vi "Periodic Tasks.vi"(8 "error in":errorcluster) -> ()   [LabVIEW 2017]
doc: "This VI runs in parallel to other tasks. It can contain as many user-defined periodic loops as you need. These can carry out PID or other sorts of timed response."
uses:
  <vilib>/Rock Robotics/WPI/DriverStation/WPI_DriverStationRobotMode2.ctl
  <vilib>/Rock Robotics/WPI/Utilities/WPI_GetSetVariantRefNum.vi
  Robot Global Data.vi
  <vilib>/Rock Robotics/Network Tables/NT Write Number.vi
panel:
  out "raw yaw":dbl
  out "original Heading":dbl
  out "ignore":dbl
  out "fused":dbl
  out "new yaw":dbl
  in  "Cluster":T1
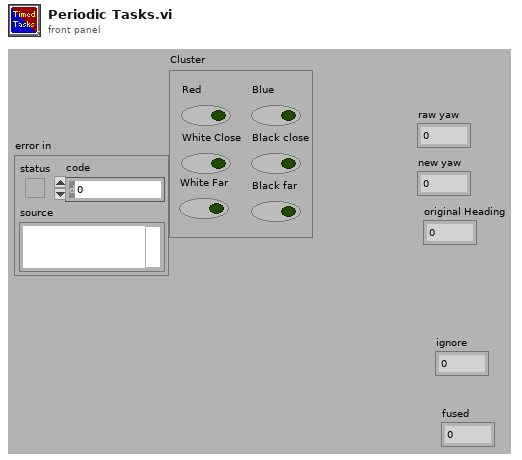
[diagram p1: front panel]
types:
  T1 = cluster{"Red":bool, "Blue":bool, "Black close":bool, "White Close":bool, "White Far":bool, "Black far":bool}
  T2 = typedef "WPI_JoystickDevRef.ctl" = cluster{"Device":T3}
  T3 = typedef "WPI_JoystickDeviceEnum.ctl" = enum16{"USB 0", "USB 1", "USB 2", "USB 3", "USB 4", "USB 5"}
  T4 = typedef "WPI_RobotDriveDevRef.ctl" = cluster{"DevStatus":errorcluster, "Motors[]":T5[], "Square Inputs":bool, "Max Output":dbl}
  T5 = typedef "WPI_MotorControlDeviceRef.ctl" = cluster{"DeviceStatus":errorcluster, "Type":T6, "PWM":cluster{"PWM Channel":T7, "DeadBand":T8}, "CAN":cluster{"Device Number":u8, "SetOutput VI Ref":variant, "GetOutput VI Ref":variant, "Enable VI Ref":variant, "Disable VI Ref":variant, "Data":variant}, "Invert":bool, "DIO PWM":cluster{"PWM \"Enable\" Channel":T7, "DIOChannel":T9, "PWM Rate":dbl}}
  T6 = typedef "WPI_MotorControlType.ctl" = enum16{"PWM", "CAN", "DIO PWM"}
  T7 = typedef "FPGA_DIOPWMChannel.ctl" = enum8{"PWM 0", "PWM 1", "PWM 2", "PWM 3", "PWM 4", "PWM 5", "PWM 6", "PWM 7", "PWM 8", "PWM 9", "PWM MXP 0", "PWM MXP 1", "PWM MXP 2", "PWM MXP 3", "PWM MXP 4", "PWM MXP 5", "PWM MXP 6", "PWM MXP 7", "PWM MXP 8", "PWM MXP 9", "Invalid"}
  T8 = typedef "WPI_PWMDeadband.ctl" = cluster{"Name":string, "maxPositivePwm":i32, "minPositivePwm":i32, "centerPwm":i32, "maxNegativePwm":i32, "minNegativePwm":i32, "angularRange":u16}
  T9 = typedef "FPGA_DIOChannel.ctl" = enum8{"DIO 0", "DIO 1", "DIO 2", "DIO 3", "DIO 4", "DIO 5", "DIO 6", "DIO 7", "DIO 8", "DIO 9", "DIO MXP 0", "DIO MXP 1", "DIO MXP 2", "DIO MXP 3", "DIO MXP 4", "DIO MXP 5", "DIO MXP 6", "DIO MXP 7", "DIO MXP 8", "DIO MXP 9", "DIO MXP 10", "DIO MXP 11", "DIO MXP 12", "DIO MXP 13", "DIO MXP 14", "DIO MXP 15", "SPI Port CS1", "SPI Port CS2", "SPI Port CS3", "SPI Port MISO", "SPI Port MOSI", "Invalid"}
  T10 = typedef "WPI_DriverStationRobotMode2.ctl" = enum16{"Autonomous Disabled", "Autonomous Enabled", "Teleop Disabled", "Teleop Enabled", "Disconnected", "Finish", "Test Disabled", "Test Enabled", "Emergency Stopped"}
  T11 = cluster{"Yaw":dbl, "Roll":dbl, "Pitch":dbl, "Heading":dbl, "Fused Heading":dbl}
  T12 = cluster{"JoystickDevRef":T2, "RobotDriveDevRef":T4}
  T13 = typedef "WPI_EncoderDevRef.ctl" = cluster{"DevStatus":errorcluster, "EncoderIndex":T14, "CounterIndex":T15, "DistancePerCount":dbl, "Decoding Type":T16}
  T14 = typedef "FPGA_EncoderIdx.ctl" = enum8{"Enc 0", "Enc 1", "Enc 2", "Enc 3", "Enc 4", "Enc 5", "Enc 6", "Enc 7", "Invalid"}
  T15 = typedef "FPGA_CounterCtrSystemIndex.ctl" = enum8{"Ctr 0", "Ctr 1", "Ctr 2", "Ctr 3", "Ctr 4", "Ctr 5", "Ctr 6", "Ctr 7", "Invalid"}
  T16 = typedef "WPI_EncoderType.ctl" = enum16{"1x", "2x", "4x"}
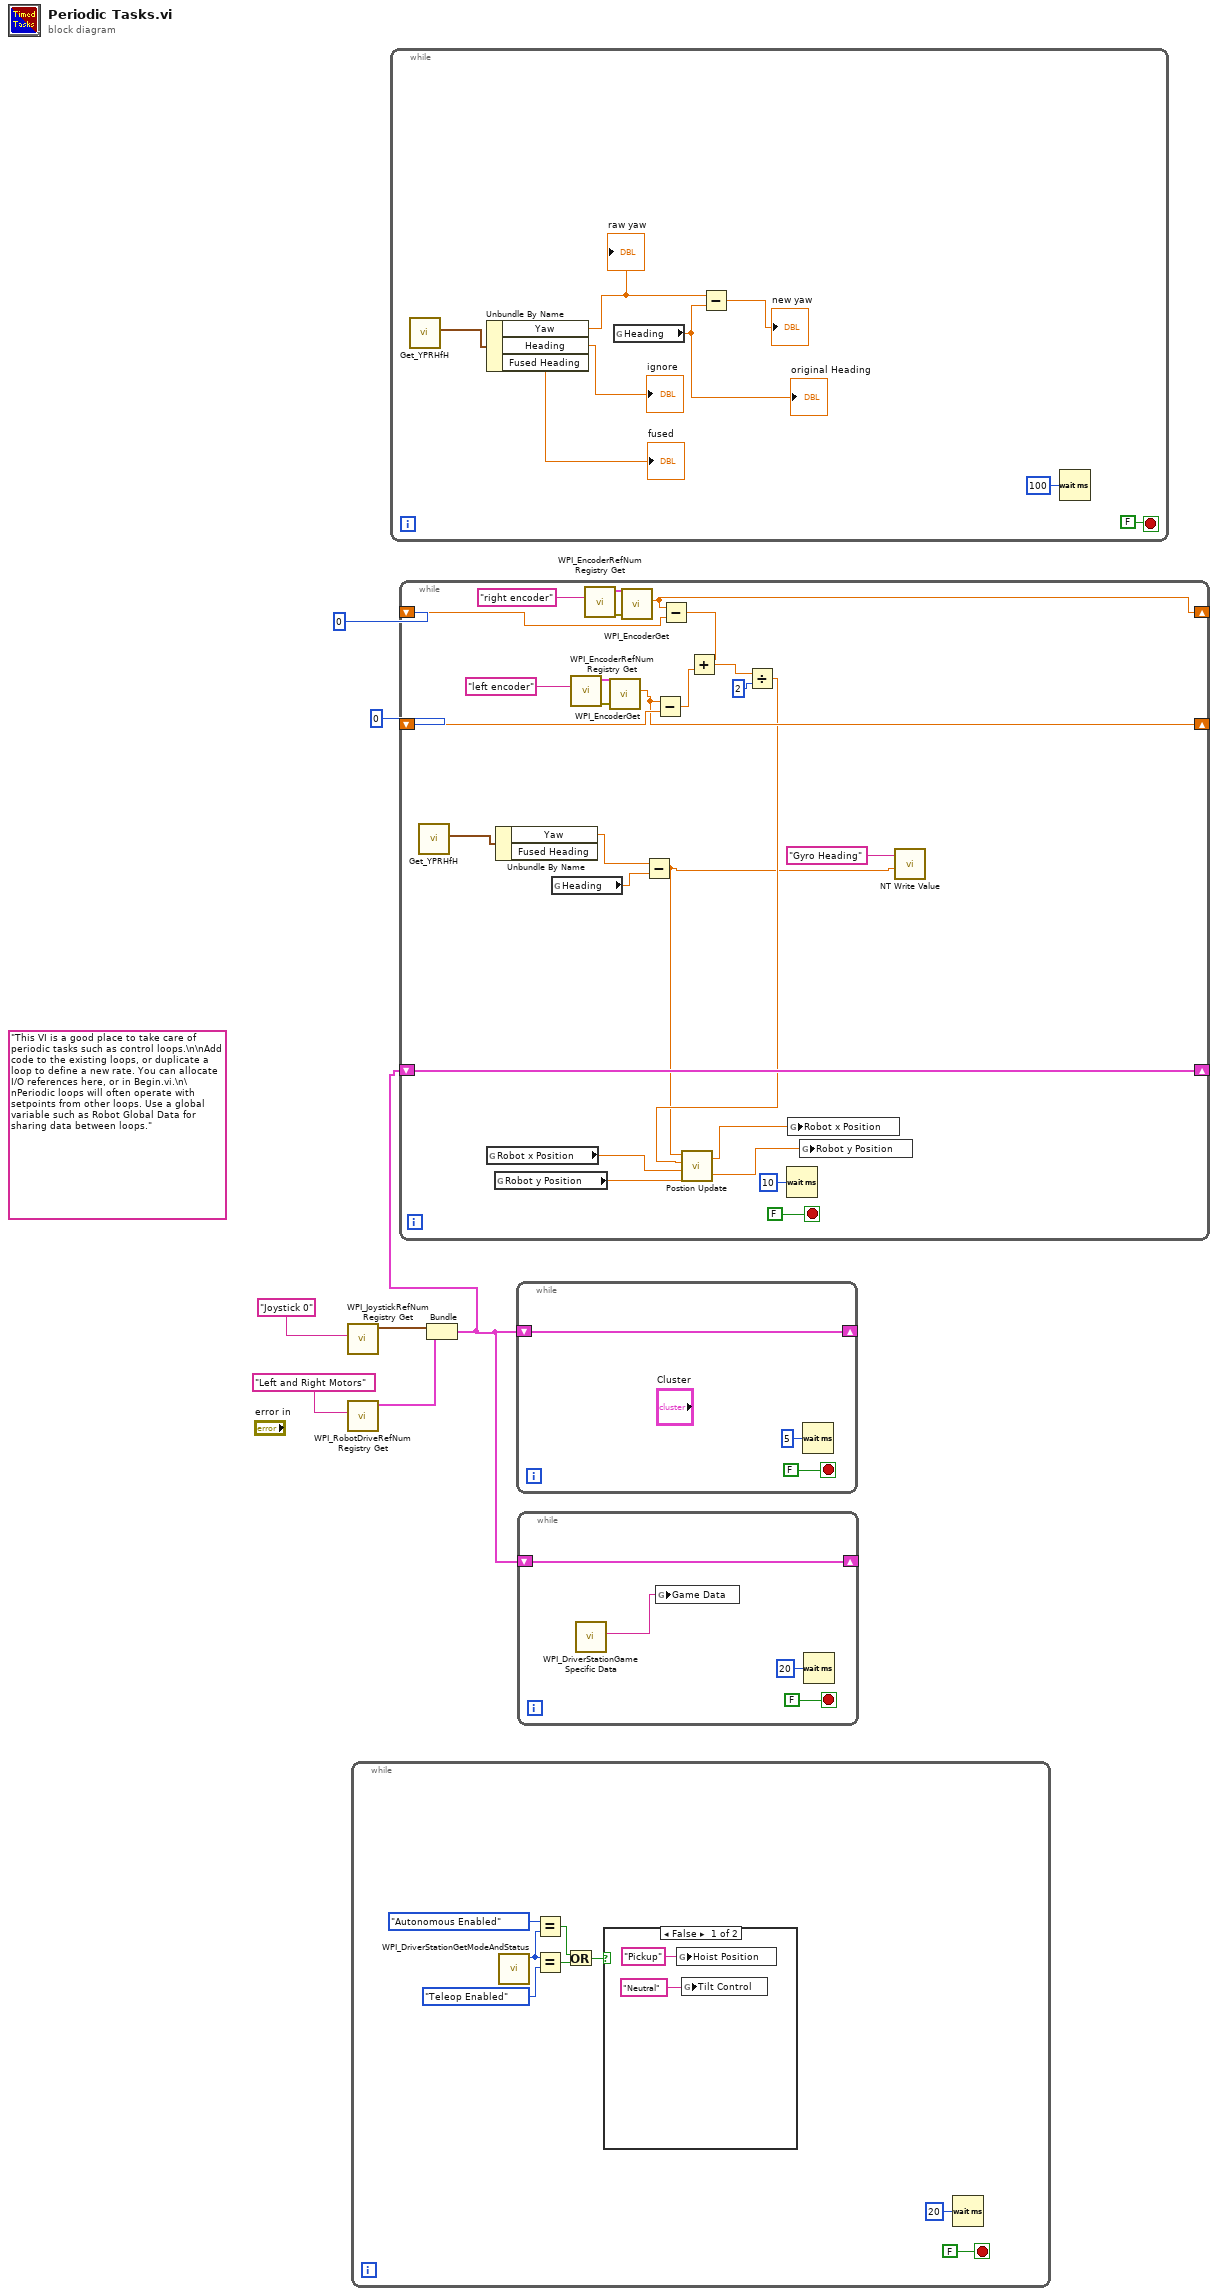
[diagram p0: block diagram]
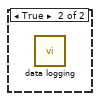
[diagram p2: hidden frame]
diagram:
  (unwired) "This VI is a good place to take care of periodic tasks such as control loops.\n\nAdd code to the existing loops, or duplicate a loop to define a new rate. You can allocate I/O references here, or in Begin.vi.\n\nPeriodic loops will often operate with setpoints from other loops. Use a global variable such as Robot Global Data for sharing data between loops."
  n1 = call <vilib>:"WPI_JoystickRefNum Registry Get.vi"("refnum name"="Joystick 0") -> ("JoystickDevRef"=w5:T2)  [unwired: 1 in, 9 out]
  n2 = call <vilib>:"WPI_RobotDriveRefNum Registry Get.vi"("refnum name"="Left and Right Motors") -> ("RobotDriveDevRef"=w4:T4)  [unwired: 1 in, 9 out]
  n3 = while {
    stop <- FALSE stop-if-true
    n4 = call <vilib>:"WPI_DriverStationGetModeAndStatus.vi"() -> ("Robot Mode"=w13:T10)  [unwired: 10 in, 1 out]
    n5 = Equal?(x=WPI_DriverStationRobotMode2."Autonomous Enabled", y=w13) -> (x = y?=w10:bool)
    n6 = Equal?(x=w13, y=WPI_DriverStationRobotMode2."Teleop Enabled") -> (x = y?=w11:bool)
    n7 = Or(x=w10, y=w11) -> (x .or. y?=w9:bool)
    n8 = case shown="False" w9 {
      frame False {
        n9 = global write "Robot Global Data.vi" "Hoist Position"("Pickup" ("Game Data")) -> ()
        n10 = global write "Robot Global Data.vi" "Tilt Control"("Neutral") -> ()
      }
      frame True {
        n11 = call "data logging.vi"() -> ()  [unwired: 12 in]
      }
    }
    n12 = Wait (ms)(milliseconds to wait=u32 20) -> ()  [unwired: 1 out]
  }
  n13 = while {
    stop <- FALSE stop-if-true
    n14 = call <vilib>:"Get_YPRHfH.vi"() -> ("YRPHfH"=w25:T11)  [unwired: 11 in]
    n15 = Unbundle By Name(w25) -> ("Yaw"=w18:dbl, "Heading"=→"ignore":dbl, "Fused Heading"=→"fused":dbl)
    "raw yaw" <- w18
    n16 = global read "Robot Global Data.vi" "Heading"() -> (w19:dbl)
    "original Heading" <- w19
    n17 = Subtract(x=w18, y=w19) -> (x-y=→"new yaw":dbl)
    n18 = Wait (ms)(milliseconds to wait=u32 100) -> ()  [unwired: 1 out]
  }
  n19 = Bundle("JoystickDevRef"=w5, "RobotDriveDevRef"=w4) -> (w1:T12)  [unwired: 1 out]
  n20 = while {
    shift-right: [w50] -> _
    shift-left: w1 -> [w50]
    shift-right: [w35] -> _
    shift-left: 0 -> [w40]
    shift-right: [w36] -> _
    shift-left: 0 -> [w38]
    stop <- FALSE stop-if-true
    n21 = call <vilib>:"Get_YPRHfH.vi"() -> ("YRPHfH"=w37:T11)  [unwired: 11 in]
    n22 = global read "Robot Global Data.vi" "Robot x Position"() -> (w31:dbl)
    n23 = global read "Robot Global Data.vi" "Robot y Position"() -> (w30:dbl)
    n24 = Unbundle By Name(w37) -> ("Yaw"=w34:dbl)  [unwired: 1 out]
    n25 = global read "Robot Global Data.vi" "Heading"() -> (w33:dbl)
    n26 = call <vilib>:"WPI_EncoderRefNum Registry Get.vi"("refnum name"="left encoder") -> ("error out"=w47:errorcluster, "EncoderDevRef"=w46:T13)  [unwired: 9 in]
    n27 = call <vilib>:"WPI_EncoderRefNum Registry Get.vi"("refnum name"="right encoder") -> ("error out"=w49:errorcluster, "EncoderDevRef"=w48:T13)  [unwired: 9 in]
    n28 = call <vilib>:"WPI_EncoderGet.vi"("error in (no error)"=w47, "EncoderDevRef"=w46) -> ("Distance"=w35:dbl)  [unwired: 4 in, 5 out]
    n29 = call <vilib>:"WPI_EncoderGet.vi"("error in (no error)"=w49, "EncoderDevRef"=w48) -> ("Distance"=w36:dbl)  [unwired: 4 in, 5 out]
    n30 = Subtract(x=w34, y=w33) -> (x-y=w26:dbl)
    n31 = Subtract(x=w35, y=w40) -> (x-y=w41:dbl)
    n32 = Subtract(x=w36, y=w38) -> (x-y=w39:dbl)
    n33 = Add(x=w39, y=w41) -> (x+y=w43:dbl)
    n34 = Divide(x=w43, y=2) -> (x/y=w32:dbl)
    n35 = call "Postion Update.vi"("Y position in"=w30, "X position in"=w31, "Distance"=w32, "Heading"=w26) -> ("Y position"=w28:dbl, "X position"=w29:dbl)
    n36 = Wait (ms)(milliseconds to wait=u32 10) -> ()  [unwired: 1 out]
    n37 = global write "Robot Global Data.vi" "Robot x Position"(w29) -> ()
    n38 = global write "Robot Global Data.vi" "Robot y Position"(w28) -> ()
    n39 = call-poly <vilib>:"NT Write Value.vi"("Numeric"=w26, "Name"="Gyro Heading") -> ()  [unwired: 9 in, 1 out]
  }
  n40 = while {
    shift-right: [w53] -> _
    shift-left: w1 -> [w53]
    stop <- FALSE stop-if-true
    n41 = Wait (ms)(milliseconds to wait=u32 5) -> ()  [unwired: 1 out]
  }
  n42 = while {
    shift-right: [w57] -> _
    shift-left: w1 -> [w57]
    stop <- FALSE stop-if-true
    n43 = call <vilib>:"WPI_DriverStationGame Specific Data.vi"() -> ("Game Specific Data"=w56:string)  [unwired: 11 in]
    n44 = global write "Robot Global Data.vi" "Game Data"(w56) -> ()
    n45 = Wait (ms)(milliseconds to wait=u32 20) -> ()  [unwired: 1 out]
  }
